vi "seek_tag.vi"(8 "error in":errorcluster, 10 "Name":string, 11 "refnum":refnum<file>) -> (0 "error out":errorcluster, 2 "error":string, 3 "refnum":refnum<file>)   [LabVIEW 2012]
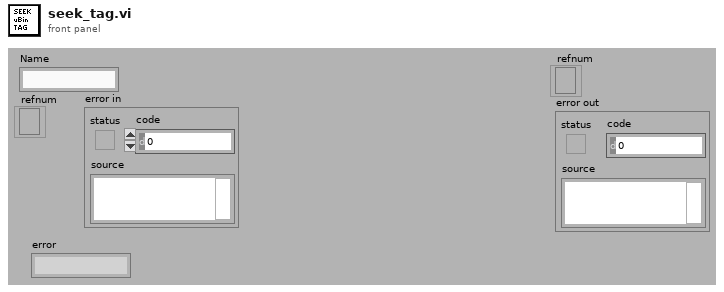
[diagram p1: front panel]
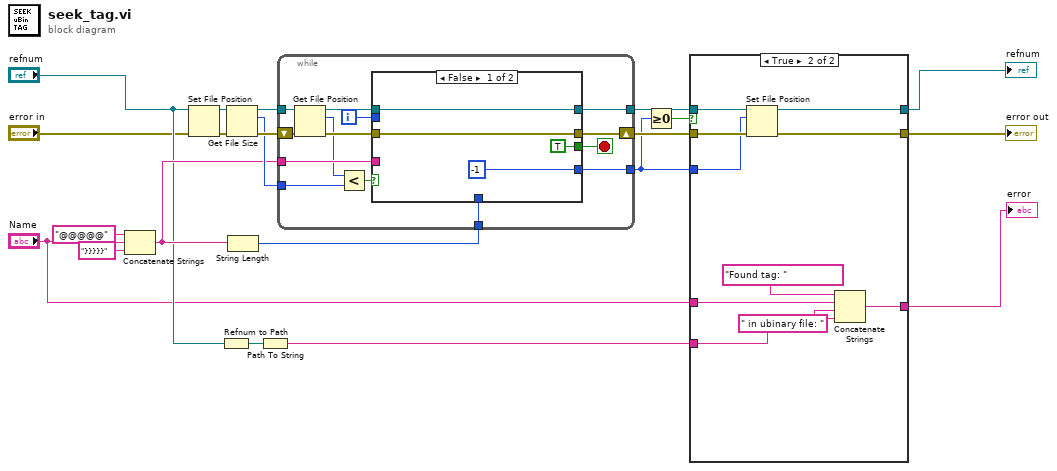
[diagram p0: block diagram]
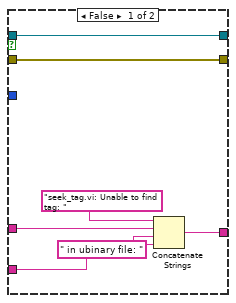
[diagram p2: hidden frame]
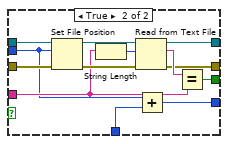
[diagram p3: hidden frame]
diagram:
  n1 = Concatenate Strings("@@@@@" ("string"), "Name", "}}}}}" ("string")) -> (w9:string)
  n2 = Set File Position(refnum="refnum", error in="error in") -> (refnum out=w5:refnum<file>, error out=w3:errorcluster)  [unwired: 2 in]
  n3 = Refnum to Path(1:"refnum") -> (0:w8:path)
  n4 = Get File Size(file=w5, error in=w3) -> (refnum out=w15:refnum<file>, size (in bytes)=w13:i64, 0:w14:errorcluster)
  n5 = String Length(string=w9) -> (length=w12:i32)
  n6 = Path To String(path=w8) -> (string=w1:string)
  n7 = while {
    tunnel: w15 -> [w31]
    shift-right: [w33] -> w21
    shift-left: w14 -> [w29]
    tunnel: w9 -> [w35]
    tunnel: [w32] -> w20
    tunnel: [w23] -> w10
    tunnel: w13 -> [w26]
    tunnel: w12 -> [w22]
    i -> [w24]
    stop <- w34 stop-if-true
    n8 = Get File Position(4:w29, 7:w31) -> (0:w28:errorcluster, 2:w27:i64, 3:w30:refnum<file>)
    n9 = Less?(x=w27, y=w26) -> (x < y?=w25:bool)
    n10 = case shown="False" w25 {
      tunnel: w35 -> [_ w48]
      tunnel: [TRUE w47] -> w34
      tunnel: [w37 w46] -> w33
      tunnel: [w38 w45] -> w32
      tunnel: w24 -> [_ w41]
      tunnel: w30 -> [w38 w44]
      tunnel: w28 -> [w37 w43]
      tunnel: [-1 ("x") w40] -> w23
      tunnel: w22 -> [_ w42]
      frame False {
      }
      frame True {
        n11 = Set File Position(offset (in bytes) (0)=w41, refnum=w44, error in=w43) -> (refnum out=w52:refnum<file>, error out=w50:errorcluster)  [unwired: 1 in]
        n12 = String Length(string=w48) -> (length=w51:i32)
        n13 = Read from Text File(file (use dialog)=w52, count=w51, error in=w50) -> (refnum out=w45:refnum<file>, text=w49:string, error out=w46:errorcluster)  [unwired: 1 in, 1 out]
        n14 = Add(x=w41, y=w42) -> (x+y=w40:i32)
        n15 = Equal?(x=w49, y=w48) -> (x = y?=w47:bool)
      }
    }
  }
  n16 = Greater Or Equal To 0?(x=w10) -> (x >= 0?=w11:bool)
  n17 = case shown="True" w11 {
    tunnel: w21 -> [w58 w69]
    tunnel: w20 -> [w59 w68]
    tunnel: [w59 w67] -> w19
    tunnel: [w58 w66] -> w18
    tunnel: w10 -> [_ w65]
    tunnel: [w55 w62] -> w7
    tunnel: "Name" -> [w54 w60]
    tunnel: w1 -> [w53 w61]
    frame False {
      n18 = Concatenate Strings("seek_tag.vi: Unable to find tag: " ("source"), w54, " in ubinary file: " ("string"), w53) -> (w55:string)
    }
    frame True {
      n19 = Set File Position(offset (in bytes) (0)=w65, refnum=w68, error in=w69) -> (refnum out=w67:refnum<file>, error out=w66:errorcluster)  [unwired: 1 in]
      n20 = Concatenate Strings("Found tag: " ("source"), w60, " in ubinary file: " ("string"), w61) -> (w62:string)
    }
  }
  "refnum" <- w19
  "error out" <- w18
  "error" <- w7
